vi "Keep Alive.vi"(8 "error in (no error)":errorcluster, 9 "Connection Name":string) -> (0 "error out":errorcluster)   [LabVIEW 2015, in "LabSSH.lvlib"]
uses:
  LabSSH.lvlib
  FGV State..enum.ctl
  C:/Working Folder/ssh.git/LabSSH Library/References/LabSSH.dll
  References/LabSSH.dll
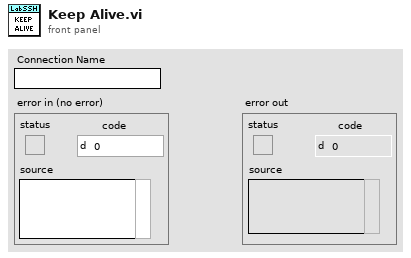
[diagram p1: front panel]
types:
  T1 = typedef "LabSSH.lvlib/FGV State..enum.ctl" = enum16{"GET", "SET"}
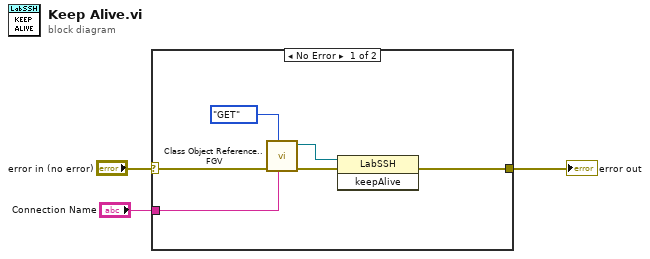
[diagram p0: block diagram]
diagram:
  n1 = case shown="No Error" "error in (no error)" {
    selector: "error in (no error)" -> [w6 w10]
    tunnel: [w5 w10] -> w2
    tunnel: "Connection Name" -> [w4 _]
    frame No Error {
      n2 = call "Class Object Reference..FGV.vi"("Connection Name"=w4, "FGV State (GET)"=FGV_State..enum."GET" ("FGV State"), "error in (no error)"=w6) -> ("error out"=w7:errorcluster, "LabSSH ref out"=w8:refnum<k24>)  [unwired: 7 in]
      n3 = invoke on="Invoke Node" class="LabSSH" method="keepAlive"(reference=w8, error in=w7) -> (error out=w5:errorcluster)  [unwired: 1 in, 2 out]
    }
    frame Error {
    }
  }
  "error out" <- w2
